vi "Set Value.vi"(7 "TOML string":string, 8 "error in (no error)":errorcluster, 9 "start position":i32, 10 "Value":T3, 11 "Context in":T2[](array[typedef])) -> (0 "error out":errorcluster, 1 "offset past match":i32, 2 "State":T1, 3 "Context out":T2[](array[typedef]))   [LabVIEW 2017, in "TOML.lvlib"]
uses:
  TOML.lvlib
  Value.ctl
  Value Type.ctl
  Context.ctl
  State.ctl
  Table Context.ctl
  Key-Value Pair.ctl
  Table Array Context.ctl
  Array Context.ctl
  <vilib>/ErrorRing/Error Ring.xnode
  <vilib>/regexp/Match Regular Expression.xnode
panel:
  in  "Define":bool=TRUE
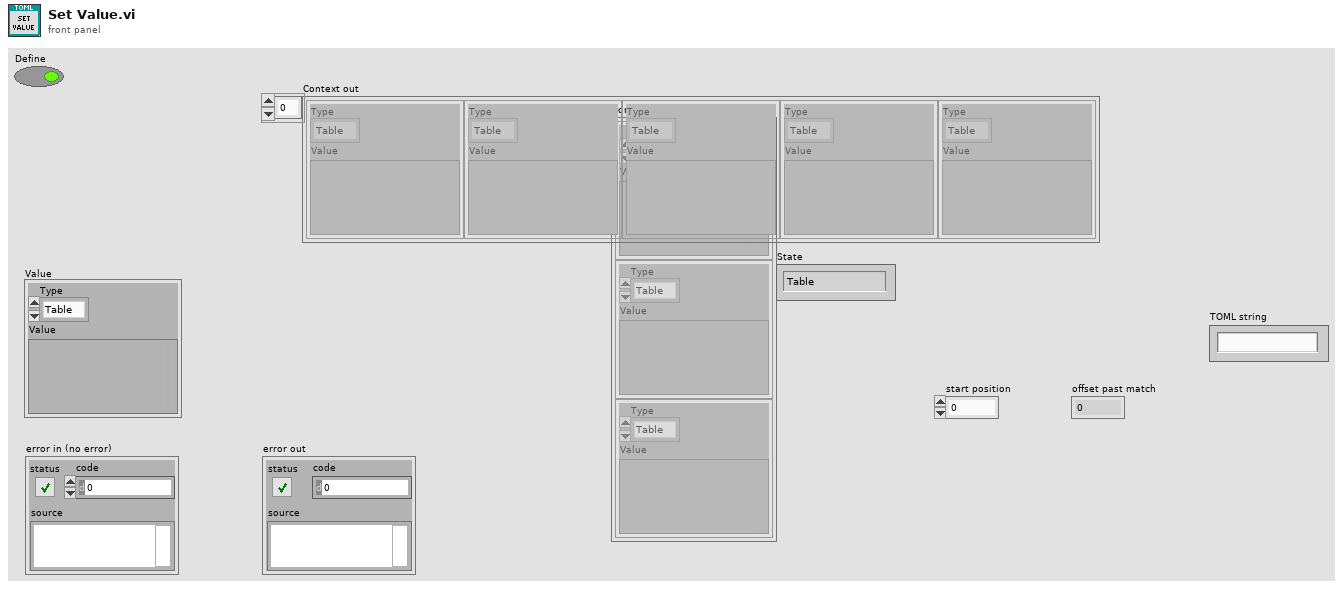
[diagram p1: front panel]
types:
  T1 = typedef "TOML.lvlib/State.ctl" = enum16{"Table", "Value", "Inline Table"}
  T2 = typedef "TOML.lvlib/Context.ctl" = cluster{"Type":enum16{"Table", "Array", "Inline Table", "Table Array"}, "Value":variant}
  T3 = typedef "TOML.lvlib/Value.ctl" = cluster{"Type":T4, "Value":variant}
  T4 = typedef "TOML.lvlib/Value Type.ctl" = enum16{"Table", "Array", "String", "Integer", "Float", "Boolean", "Offset Date-Time", "Local Date-Time", "Local Date", "Local Time", "Path"}
  T5 = typedef "TOML.lvlib/Table Context.ctl" = cluster{"Table":T6[], "Key":string, "Defined Keys":string[]}
  T6 = typedef "TOML.lvlib/Key-Value Pair.ctl" = cluster{"Key":string, "Value":T3}
  T7 = typedef "TOML.lvlib/Table Array Context.ctl" = cluster{"Table Array":cluster{"Table":T6[]}[], "Index":i32, "Key":string}
  T8 = typedef "TOML.lvlib/Array Context.ctl" = cluster{"Array":T3[], "Index":i32, "Empty":bool, "Type":T4}
  T9 = enum16{"Table", "Array", "Inline Table", "Table Array"}
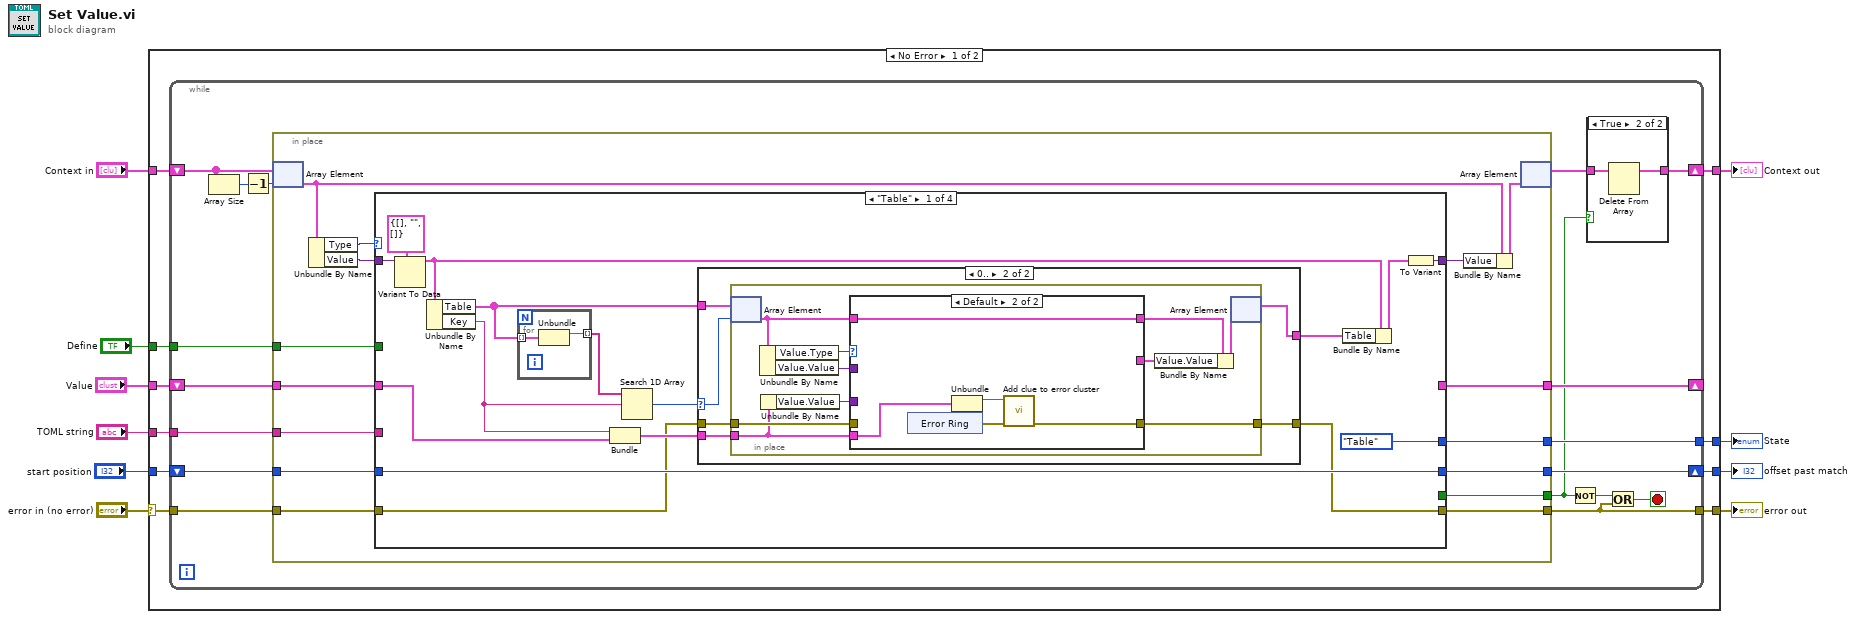
[diagram p0: block diagram]
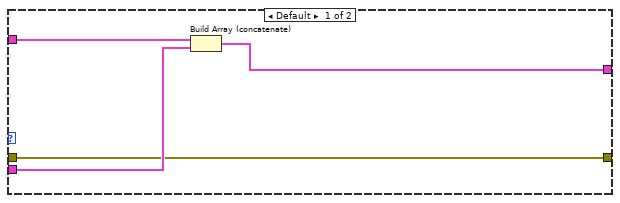
[diagram p3: hidden frame]
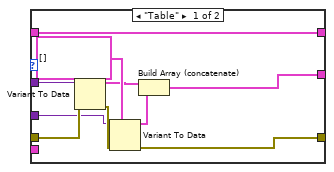
[diagram p4: hidden frame]
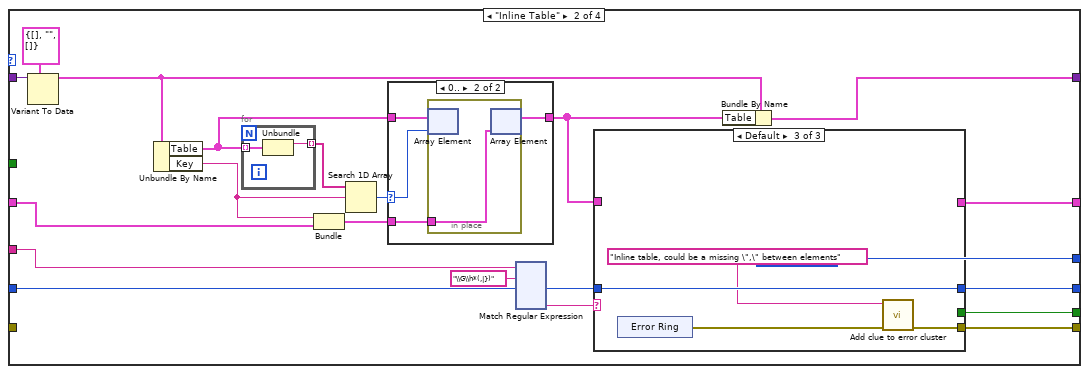
[diagram p5: hidden frame]
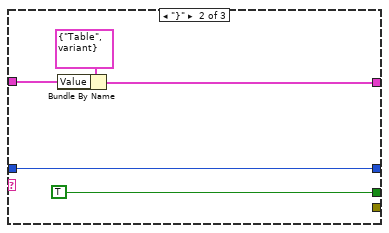
[diagram p7: hidden frame]
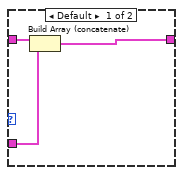
[diagram p8: hidden frame]
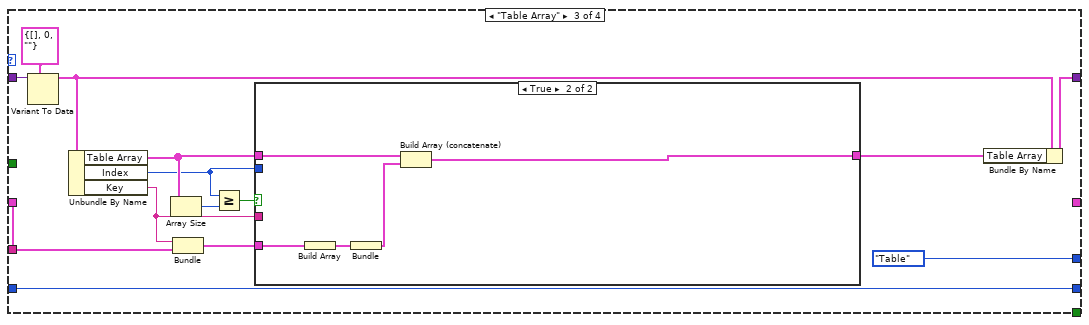
[diagram p9: hidden frame]
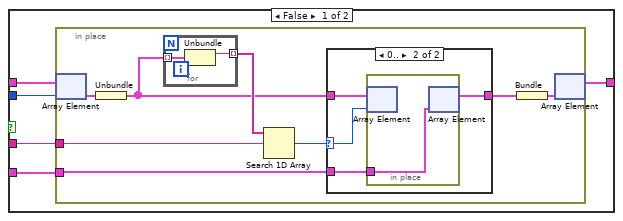
[diagram p10: hidden frame]
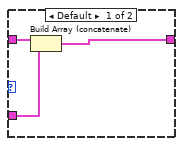
[diagram p11: hidden frame]
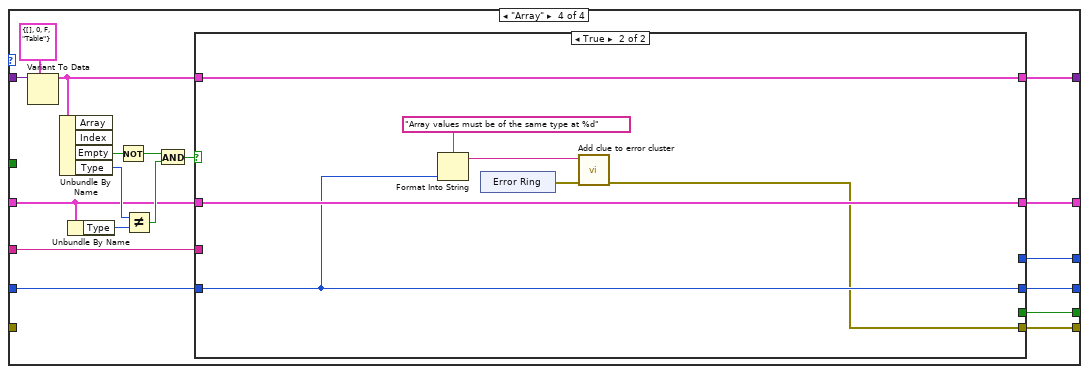
[diagram p12: hidden frame]
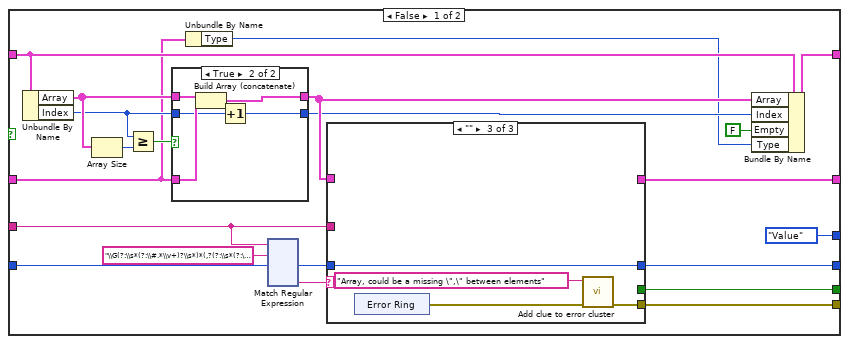
[diagram p13: hidden frame]
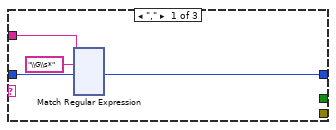
[diagram p14: hidden frame]
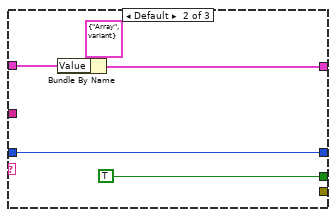
[diagram p15: hidden frame]
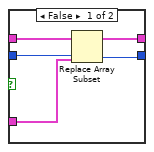
[diagram p16: hidden frame]
diagram:
  n1 = case shown="No Error" "error in (no error)" {
    selector: "error in (no error)" -> [w15 w614]
    tunnel: "Context in" -> [w20 w612]
    tunnel: [w19 w612] -> w9
    tunnel: "Value" -> [w18 _]
    tunnel: [w17 _] -> w7
    tunnel: [w16 w614] -> w6
    tunnel: "start position" -> [w14 w613]
    tunnel: "TOML string" -> [w13 _]
    tunnel: [w12 w613] -> w2
    tunnel: "Define" -> [w11 _]
    frame No Error {
      n2 = while {
        tunnel: [w33] -> w17
        tunnel: w13 -> [w28]
        shift-right: [w26] -> w12
        shift-left: w14 -> [w29]
        tunnel: w15 -> [w32]
        tunnel: [w30] -> w16
        shift-right: [w25] -> _
        shift-left: w18 -> [w34]
        shift-right: [w23] -> w19
        shift-left: w20 -> [w35]
        tunnel: w11 -> [w21]
        stop <- w31 stop-if-true
        n3 = Array Size(array=w35) -> (size(s)=w37:i32)
        n4 = Decrement(x=w37) -> (x-1=w36:i32)
        n5 = in-place {
          in-place-border: w34 -> [w50]
          in-place-border: [w49] -> w33
          in-place-border: [w48] -> w30
          in-place-border: w32 -> [w47]
          in-place-border: [w44] -> w22
          in-place-border: w29 -> [w46]
          in-place-border: w28 -> [w45]
          in-place-border: [w43] -> w25
          in-place-border: [w42] -> w26
          in-place-border: w21 -> [w41]
          n6 = in-place-array #1(w35, w36) -> (w53:T2)
          n7 = Unbundle By Name(w53) -> ("Type"=w55:T9, "Value"=w54:variant)
          n8 = case shown="\"Table\"" w55 {
            tunnel: w54 -> [w71 w130 w281 w327]
            tunnel: w50 -> [w65 w124 w277 w311]
            tunnel: [w60 w110 w270 w326] -> w52
            tunnel: [State."Table" ("State") State."Inline Table" ("State") State."Table" ("State") w324] -> w49
            tunnel: [w56 w111 _ w319] -> w48
            tunnel: w47 -> [w57 _ _ _]
            tunnel: w46 -> [w58 w120 w268 w322]
            tunnel: w45 -> [_ w119 _ w318]
            tunnel: [_ w115 _ w323] -> w44
            tunnel: [_ w113 _ w320] -> w43
            tunnel: [w58 w112 w268 w321] -> w42
            tunnel: w41 -> [_ _ _ _]
            frame "Table" {
              n9 = Variant To Data(type=T5 {"Table"=[], "Key"="", "Defined Keys"=[]} ("Table Context"), Variant=w71) -> (data=w64:T5)  [unwired: 1 in, 1 out]
              n10 = Unbundle By Name(w64) -> ("Table"=w67:T6[], "Key"=w66:string)
              n11 = for {
                tunnel: w67 -> [w109] mode=indexing
                tunnel: [w108] -> w69 mode=indexing
                n12 = Unbundle(w109) -> ("Key"=w108:string)  [unwired: 1 out]
              }
              n13 = Bundle("Key"=w66, "Value"=w65) -> (w61:cluster{"Key":string, "Value":T3})  [unwired: 1 in]
              n14 = Search 1D Array(1D array=w69, element=w66) -> (index of element=w68:i32)  [unwired: 1 in]
              n15 = case shown="0.." w68 {
                selector: w68 -> [_ w79]
                tunnel: w67 -> [w75 w81]
                tunnel: [w74 w80] -> w63
                tunnel: w61 -> [w73 w78]
                tunnel: w57 -> [w72 w77]
                tunnel: [w72 w76] -> w56
                frame Default {
                  n16 = Build Array (concatenate)(w75, w73) -> (w74:T6[])
                }
                frame 0.. {
                  n17 = in-place {
                    in-place-border: w78 -> [w84]
                    in-place-border: w77 -> [w86]
                    in-place-border: [w85] -> w76
                    n18 = in-place-array #2(w81, w79) -> (w90:T6)
                    n19 = Unbundle By Name(w90) -> ("Value.Type"=w89:T4, "Value.Value"=w88:variant)
                    n20 = Unbundle By Name(w84) -> ("Value.Value"=w83:variant)
                    n21 = case shown="Default" w89 {
                      tunnel: [w101 w106] -> w91
                      tunnel: w90 -> [w101 w106]
                      tunnel: w88 -> [w100 _]
                      tunnel: w84 -> [_ w103]
                      tunnel: w86 -> [w99 _]
                      tunnel: [w93 w104] -> w85
                      tunnel: w83 -> [w92 _]
                      tunnel: [w94 _] -> w82
                      frame "Table" {
                        w97 = T6[] []
                        n22 = Variant To Data(error in=w99, type=w97, Variant=w100) -> (data=w96:T6[], error out=w98:errorcluster)
                        n23 = Variant To Data(error in=w98, type=w97, Variant=w92) -> (data=w95:T6[], error out=w93:errorcluster)
                        n24 = Build Array (concatenate)(w96, w95) -> (w94:T6[])
                      }
                      frame Default {
                        n25 = xnode "Error Ring"() -> ("error out"=w105:errorcluster)
                        n26 = Unbundle(w103) -> ("Key"=w102:string)  [unwired: 1 out]
                        n27 = call "Add clue to error cluster.vi"("error in (no error)"=w105, "String"=w102) -> ("error out"=w104:errorcluster)  [unwired: 9 in]
                      }
                    }
                    n28 = Bundle By Name(cluster=w91, "Value.Value"=w82) -> (w87:T6)
                    n29 = in-place-array #2(w87) -> (w80:T6[])  [unwired: 1 out]
                  }
                }
              }
              n30 = Bundle By Name(cluster=w64, "Table"=w63) -> (w62:T5)
              n31 = To Variant(anything=w62) -> (Variant=w60:variant)
            }
            frame "Inline Table" {
              n32 = Variant To Data(type=T5 {"Table"=[], "Key"="", "Defined Keys"=[]} ("Table Context"), Variant=w130) -> (data=w123:T5)  [unwired: 1 in, 1 out]
              n33 = Unbundle By Name(w123) -> ("Table"=w126:T6[], "Key"=w125:string)
              n34 = for {
                tunnel: w126 -> [w267] mode=indexing
                tunnel: [w266] -> w128 mode=indexing
                n35 = Unbundle(w267) -> ("Key"=w266:string)  [unwired: 1 out]
              }
              n36 = Bundle("Key"=w125, "Value"=w124) -> (w122:cluster{"Key":string, "Value":T3})  [unwired: 1 in]
              n37 = Search 1D Array(1D array=w128, element=w125) -> (index of element=w127:i32)  [unwired: 1 in]
              n38 = case shown="0.." w127 {
                selector: w127 -> [_ w262]
                tunnel: w126 -> [w260 w264]
                tunnel: [w259 w263] -> w114
                tunnel: w122 -> [w258 w261]
                frame Default {
                  n39 = Build Array (concatenate)(w260, w258) -> (w259:T6[])
                }
                frame 0.. {
                  n40 = in-place {
                    in-place-border: w261 -> [w265]
                    n41 = in-place-array #3(w264, w262) -> ()  [unwired: 1 out]
                    n42 = in-place-array #3(w265) -> (w263:T6[])  [unwired: 1 out]
                  }
                }
              }
              n43 = xnode "Match Regular Expression"("input string"=w119, "regular expression"="\\G\\h*(,|})", "offset (0)"=w120) -> ("offset past match"=w116:i32, "submatch 1"=w117:string)  [unwired: 3 in, 4 out]
              n44 = case shown="Default" w117 {
                tunnel: w116 -> [w247 w248 w256]
                tunnel: [_ TRUE _] -> w115
                tunnel: w114 -> [_ w250 _]
                tunnel: [_ w249 _] -> w113
                tunnel: [w247 w248 w256] -> w112
                tunnel: [_ _ w254] -> w111
                frame "," {
                }
                frame "}" {
                  n45 = Bundle By Name(cluster=T3 {"Type"=enum."Table", "Value"=variant} ("Value"), "Value"=w250) -> (w249:T3)
                }
                frame Default {
                  n46 = xnode "Error Ring"() -> ("error out"=w255:errorcluster)
                  n47 = call "Add clue to error cluster.vi"("error in (no error)"=w255, "String"="Inline table, could be a missing \",\" between elements" ("regular expression")) -> ("error out"=w254:errorcluster)  [unwired: 9 in]
                }
              }
              n48 = Bundle By Name(cluster=w123, "Table"=w114) -> (w110:T5)
            }
            frame "Table Array" {
              n49 = Variant To Data(type=T7 {"Table Array"=[], "Index"=0, "Key"=""} ("Table Array Context"), Variant=w281) -> (data=w274:T7)  [unwired: 1 in, 1 out]
              n50 = Unbundle By Name(w274) -> ("Table Array"=w275:cluster{"Table":T6[]}[], "Index"=w272:i32, "Key"=w271:string)
              n51 = Array Size(array=w275) -> (size(s)=w279:i32)
              n52 = Bundle("Key"=w271, "Value"=w277) -> (w276:cluster{"Key":string, "Value":T3})  [unwired: 1 in]
              n53 = Greater Or Equal?(x=w272, y=w279) -> (x >= y?=w278:bool)
              n54 = case shown="True" w278 {
                tunnel: w276 -> [w283 w309]
                tunnel: w275 -> [w286 w307]
                tunnel: [w282 w305] -> w273
                tunnel: w272 -> [w285 _]
                tunnel: w271 -> [w284 _]
                frame False {
                  n55 = in-place {
                    in-place-border: w284 -> [w289]
                    in-place-border: w283 -> [w288]
                    n56 = in-place-array #4(w286, w285) -> (w294:cluster{"Table":T6[]})
                    n57 = Unbundle(w294) -> ("Table"=w290:T6[])
                    n58 = for {
                      tunnel: w290 -> [w304] mode=indexing
                      tunnel: [w303] -> w292 mode=indexing
                      n59 = Unbundle(w304) -> ("Key"=w303:string)  [unwired: 1 out]
                    }
                    n60 = Search 1D Array(1D array=w292, element=w289) -> (index of element=w291:i32)  [unwired: 1 in]
                    n61 = case shown="0.." w291 {
                      selector: w291 -> [_ w299]
                      tunnel: w290 -> [w297 w301]
                      tunnel: [w296 w300] -> w287
                      tunnel: w288 -> [w295 w298]
                      frame Default {
                        n62 = Build Array (concatenate)(w297, w295) -> (w296:T6[])
                      }
                      frame 0.. {
                        n63 = in-place {
                          in-place-border: w298 -> [w302]
                          n64 = in-place-array #5(w301, w299) -> ()  [unwired: 1 out]
                          n65 = in-place-array #5(w302) -> (w300:T6[])  [unwired: 1 out]
                        }
                      }
                    }
                    n66 = Bundle("Table"=w287) -> (w293:cluster{"Table":T6[]})  [unwired: 1 in]
                    n67 = in-place-array #4(w293) -> (w282:cluster{"Table":T6[]}[])  [unwired: 1 out]
                  }
                }
                frame True {
                  n68 = Build Array(w309) -> (w308:cluster{"Key":string, "Value":T3}[])
                  n69 = Bundle(w308) -> (w306:cluster{cluster{"Key":string, "Value":T3}[]})  [unwired: 1 in]
                  n70 = Build Array (concatenate)(w307, w306) -> (w305:cluster{"Table":T6[]}[])
                }
              }
              n71 = Bundle By Name(cluster=w274, "Table Array"=w273) -> (w270:T7)
            }
            frame "Array" {
              n72 = Variant To Data(type=T8 {"Array"=[], "Index"=0, "Empty"=FALSE, "Type"=enum."Table"} ("Array Context"), Variant=w327) -> (data=w312:T8)  [unwired: 1 in, 1 out]
              n73 = Unbundle By Name(w312) -> ("Empty"=w317:bool, "Type"=w315:T4)  [unwired: 2 out]
              n74 = Unbundle By Name(w311) -> ("Type"=w316:T4)
              n75 = Not(x=w317) -> (.not. x?=w314:bool)
              n76 = Not Equal?(x=w315, y=w316) -> (x != y?=w313:bool)
              n77 = And(x=w314, y=w313) -> (x .and. y?=w310:bool)
              n78 = case shown="True" w310 {
                tunnel: [w346 w610] -> w326
                tunnel: [State."Value" ("State") _] -> w324
                tunnel: [w340 _] -> w323
                tunnel: w322 -> [w339 w607]
                tunnel: [w338 w607] -> w321
                tunnel: [w337 w609] -> w320
                tunnel: [w336 w604] -> w319
                tunnel: w318 -> [w334 _]
                tunnel: w312 -> [w332 w610]
                tunnel: w311 -> [w329 w609]
                frame False {
                  n79 = Unbundle By Name(w332) -> ("Array"=w331:T3[], "Index"=w330:i32)
                  n80 = Array Size(array=w331) -> (size(s)=w348:i32)
                  n81 = Greater Or Equal?(x=w330, y=w348) -> (x >= y?=w347:bool)
                  n82 = case shown="True" w347 {
                    tunnel: w331 -> [w598 w603]
                    tunnel: [w596 w602] -> w341
                    tunnel: w330 -> [w595 w600]
                    tunnel: w329 -> [w597 w601]
                    tunnel: [w595 w599] -> w335
                    frame False {
                      n83 = Replace Array Subset(array=w598, new element=w597, index=w595) -> (w596:T3[])
                    }
                    frame True {
                      n84 = Build Array (concatenate)(w603, w601) -> (w602:T3[])
                      n85 = Increment(x=w600) -> (x+1=w599:i32)
                    }
                  }
                  n86 = Unbundle By Name(w329) -> ("Type"=w328:T4)
                  n87 = xnode "Match Regular Expression"("input string"=w334, "regular expression"="\\G(?:\\s*(?:\\#.*\\v+)?\\s*)*(,?(?:\\s*(?:\\#.*\\v+)?\\s*)*\\]|,)", "offset (0)"=w339) -> ("offset past match"=w342:i32, "submatch 1"=w343:string)  [unwired: 3 in, 4 out]
                  n88 = case shown="\"\"" w343 {
                    tunnel: w342 -> [w466 w585 w593]
                    tunnel: [_ TRUE _] -> w340
                    tunnel: w341 -> [_ w587 _]
                    tunnel: [_ w586 _] -> w337
                    tunnel: [w465 w585 w593] -> w338
                    tunnel: [_ _ w591] -> w336
                    tunnel: w334 -> [w467 _ _]
                    frame "," {
                      n89 = xnode "Match Regular Expression"("input string"=w467, "regular expression"="\\G\\s*", "offset (0)"=w466) -> ("offset past match"=w465:i32)  [unwired: 3 in, 5 out]
                    }
                    frame Default {
                      n90 = Bundle By Name(cluster=T3 {"Type"=enum."Array", "Value"=variant} ("Value"), "Value"=w587) -> (w586:T3)
                    }
                    frame "" {
                      n91 = xnode "Error Ring"() -> ("error out"=w592:errorcluster)
                      n92 = call "Add clue to error cluster.vi"("error in (no error)"=w592, "String"="Array, could be a missing \",\" between elements" ("regular expression")) -> ("error out"=w591:errorcluster)  [unwired: 9 in]
                    }
                  }
                  n93 = Bundle By Name(cluster=w332, "Array"=w341, "Index"=w335, "Empty"=FALSE, "Type"=w328) -> (w346:T8)
                }
                frame True {
                  n94 = Format Into String(format string="Array values must be of the same type at %d", w607) -> (resulting string=w606:string)  [unwired: 2 in, 1 out]
                  n95 = xnode "Error Ring"() -> ("error out"=w605:errorcluster)
                  n96 = call "Add clue to error cluster.vi"("error in (no error)"=w605, "String"=w606) -> ("error out"=w604:errorcluster)  [unwired: 9 in]
                }
              }
            }
          }
          n97 = Bundle By Name(cluster=w53, "Value"=w52) -> (w51:T2)
          n98 = in-place-array #1(w51) -> (w24:T2[])  [unwired: 1 out]
        }
        n99 = Not(x=w22) -> (.not. x?=w27:bool)
        n100 = case shown="True" w22 {
          tunnel: w24 -> [w38 w40]
          tunnel: [w38 w39] -> w23
          frame False {
          }
          frame True {
            n101 = Delete From Array(array=w40) -> (array with subset deleted=w39:T2[])  [unwired: 2 in, 1 out]
          }
        }
        n102 = Or(x=w27, y=w30) -> (x .or. y?=w31:bool)
      }
    }
    frame Error {
    }
  }
  "error out" <- w6
  "Context out" <- w9
  "State" <- w7
  "offset past match" <- w2
